vi "NI VeriStand - Get Item Reference by Name.vi"(8 "error in (no error)":errorcluster, 10 "Item Name":string, 11 "Parent Ref in":T1 format="%.0x") -> (0 "error out":errorcluster, 2 "Item Ref":T1 format="%.0x", 3 "Parent Ref out":T1 format="%.0x", 4 "Found":bool)   [LabVIEW 2020, in "Custom Device API.lvlib"]
doc: "Searches for <B>Item Name</B> in the device or section specified by <B>Parent Ref in</B> and, if found, returns a reference to the item."
uses:
  <vilib>/NI VeriStand/Custom Device API/Custom Device API.lvlib
  <vilib>/NI VeriStand/Custom Device API/Custom Device Item Ref.ctl
  974ee1f2-157f-4a22-b4f2-d2483865be3f.vi
  <vilib>/NI VeriStand/Custom Device API/Custom Device Offline Path.vi
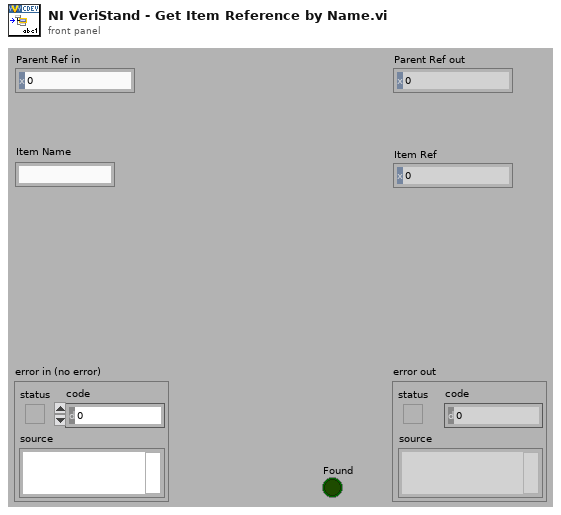
[diagram p1: front panel]
types:
  T1 = typedef "Custom Device API.lvlib/Custom Device Item Ref.ctl" = u64
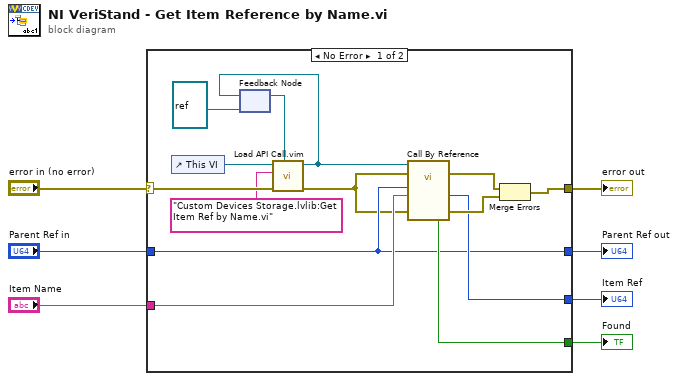
[diagram p0: block diagram]
diagram:
  n1 = case shown="No Error" "error in (no error)" {
    selector: "error in (no error)" -> [w13 w23]
    tunnel: [w20 w23] -> w7
    tunnel: "Parent Ref in" -> [w16 w22]
    tunnel: "Item Name" -> [w19 _]
    tunnel: [w16 w22] -> w4
    tunnel: [w18 _] -> w3
    tunnel: [w17 _] -> w2
    frame No Error {
      n2 = control-ref of="This VI"() -> (w14:refnum<vi>)
      n3 = feedback #1(refnum<vi> refnum ("type specifier VI Refnum (for type only)")) -> (w15:refnum<vi>)
      n4 = call "Load API Call.vim"("VI reference in"=w15, "error in (no error)"=w13, "VI qualified name"="Custom Devices Storage.lvlib:Get Item Ref by Name.vi", "Caller VI ref"=w14) -> ("error out"=w9:errorcluster, "VI reference"=w12:refnum<vi>)  [unwired: 6 in]
      n5 = feedback-in #1(w12) -> ()
      n6 = call-by-ref "?"(reference=w12, error in=w9, 8:"error in (no error)"=w9, "Item Name"=w19, "Parent Ref in"=w16) -> (error out=w8:errorcluster, 0:"error out"=w21:errorcluster, "Item Ref"=w18:T1, "Found"=w17:bool)  [unwired: 5 in, 2 out]
      n7 = Merge Errors(w8, w21) -> (w20:errorcluster)
    }
    frame Error {
    }
  }
  "Parent Ref out" <- w4
  "error out" <- w7
  "Found" <- w2
  "Item Ref" <- w3
